vi "marshalling.vi"(8 "error in (no error)":errorcluster, 10 "Variant":variant, 11 "Serializer in":refnum<class "Serializer.LV-TOML.lvclass">) -> (0 "error out":errorcluster, 2 "String":string, 3 "Serializer":refnum<class "Serializer.LV-TOML.lvclass">)   [LabVIEW 2020, in "OpenSerializer.LV-TOML.lvlib" / "Serializer.LV-TOML.lvclass"]
uses:
  Serializer.LV-TOML.lvclass
  <userlib>/LV-TOML/lib/LV-TOML.lvlib
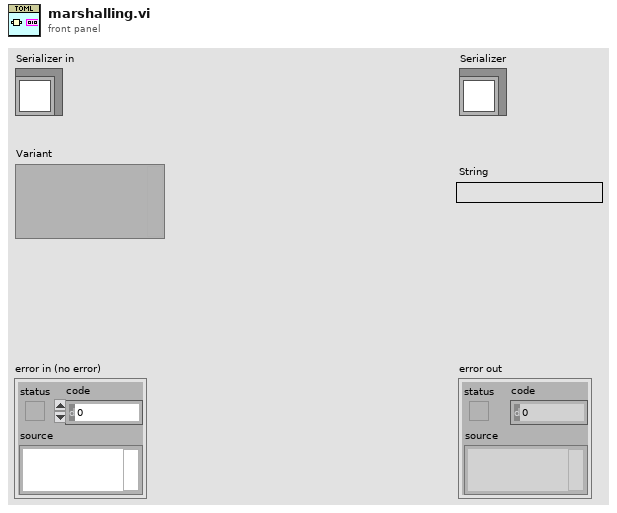
[diagram p1: front panel]
types:
  T1 = typedef "LV-TOML.lvlib/TOML Value.ctl" = cluster{"type":enum16{"Table", "Array", "String", "Integer", "Float", "Boolean", "Offset Date-Time", "Local Date-Time", "Local Date", "Local Time"}, "value":variant}
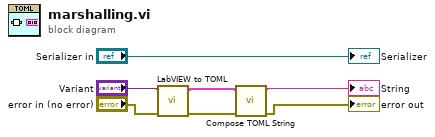
[diagram p0: block diagram]
diagram:
  n1 = call <userlib>:"LabVIEW to TOML.vi"("error in (no error)"="error in (no error)", "LV Value"="Variant") -> ("error out"=w4:errorcluster, "TOML Value"=w1:T1)  [unwired: 8 in]
  n2 = call <userlib>:"Compose TOML String.vi"("error in (no error)"=w4, "Value"=w1) -> ("error out"=→"error out":errorcluster, "String"=→"String":string)  [unwired: 8 in]
  "Serializer" <- "Serializer in"
